vi "StartupWizard.vi"() -> (0 "Exit?":bool)   [LabVIEW 2017]
uses:
  Projekt-RubikLibrary/RubikLibrary.lvlib
  Projekt-RubikLibrary/ServoEnumControl.ctl
  Projekt-RubikLibrary/ServoAbsAngleControl.ctl
panel:
  in  "Tab Control":T1(tab)
  in  "Cancel Tab1":bool
  in  "Next Tab1":bool
  in  "Cancel Tab2":bool
  in  "Back Tab2":bool
  in  "Next Tab2":bool
  in  "Next Tab3":bool
  in  "Back Tab3":bool
  in  "Cancel Tab3":bool
  in  "Cancel Tab4":bool
  in  "Back Tab4":bool
  in  "Next Tab4":bool
  in  "Back Tab5":bool
  in  "Exit":bool
  in  "Cancel Tab5":bool
  # "Start Rubik's Cube Init"
  # "Turn Front Servo to -90° (horizontal), Left and Right Servos to 0° (vertical)\n\nClick \"Do&Next >\" or Return key"
  # "Grip Left"
  # "Left Grip will close and hold the cube. \n\nClick \"Next >\" or Return key"
  # "Grip Right"
  # "Right Grip will close and hold the cube. \n\nClick \"Next >\" or Return key"
  # "Grip Front"
  # "Front Grip will close and hold the cube. \n\nClick \"Next >\" or Return key"
  # "Startup Finished?"
  # "Either\nclick \"< Back\" to go back,\nclick \"Cancel\" to abort Startup.\nclick \"Exit\" to succesfully terminate Startup."
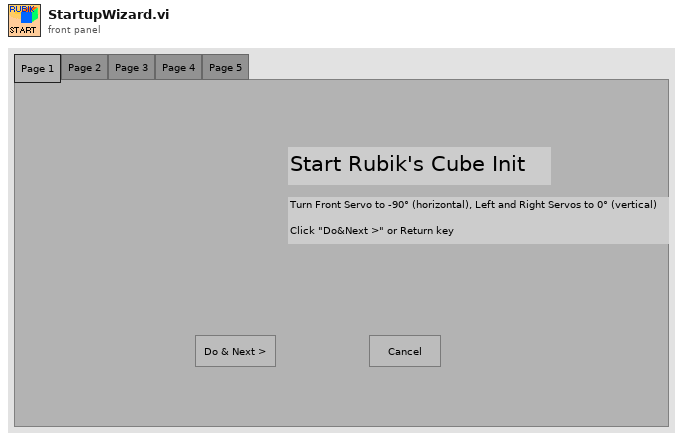
[diagram p1: front panel]
types:
  T1 = enum32{"Page 1", "Page 2", "Page 3", "Page 4", "Page 5"}
  T2 = typedef "RubikLibrary.lvlib/ServoEnumControl.ctl" = enum16{"Left Servo", "Front Servo", "Right Servo"}
  T3 = typedef "RubikLibrary.lvlib/ServoAbsAngleControl.ctl" = enum16{"-90°", "0°", "+90°"}
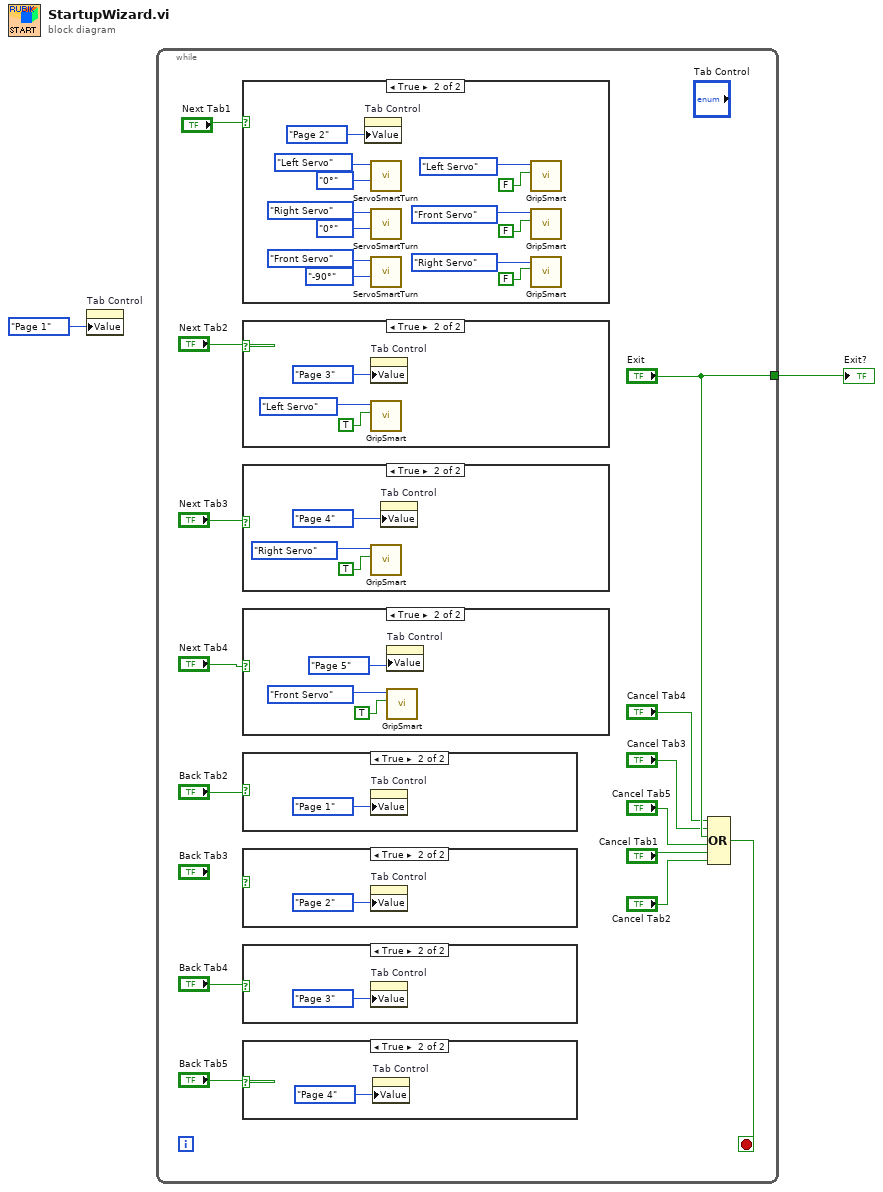
[diagram p0: block diagram]
diagram:
  n1 = property on="Tab Control" class="TabCtl (strict)"("Value"=enum32{"Page 1", "Page 2", "Page 3"}."Page 1" ("Tab Control")) -> ()  [unwired: 2 in, 2 out]
  n2 = while {
    tunnel: ["Exit"] -> w1
    stop <- w14 stop-if-true
    n3 = case shown="True" "Next Tab1" {
      frame False {
      }
      frame True {
        n4 = property on="Tab Control" class="TabCtl (strict)"("Value"=enum32{"Page 1", "Page 2", "Page 3"}."Page 2" ("Tab Control")) -> ()  [unwired: 2 in, 2 out]
        n5 = call "ServoSmartTurn.vi"("Turn to (in)"=ServoAbsAngleControl."0°", "Servo"=ServoEnumControl."Left Servo") -> ()  [unwired: 8 in, 2 out]
        n6 = call "ServoSmartTurn.vi"("Turn to (in)"=ServoAbsAngleControl."0°", "Servo"=ServoEnumControl."Right Servo") -> ()  [unwired: 8 in, 2 out]
        n7 = call "ServoSmartTurn.vi"("Turn to (in)"=ServoAbsAngleControl."-90°", "Servo"=ServoEnumControl."Front Servo") -> ()  [unwired: 8 in, 2 out]
        n8 = call "GripSmart.vi"("Turn to (in)"=FALSE, "Servo"=ServoEnumControl."Left Servo") -> ()  [unwired: 8 in, 2 out]
        n9 = call "GripSmart.vi"("Turn to (in)"=FALSE, "Servo"=ServoEnumControl."Front Servo") -> ()  [unwired: 8 in, 2 out]
        n10 = call "GripSmart.vi"("Turn to (in)"=FALSE, "Servo"=ServoEnumControl."Right Servo") -> ()  [unwired: 8 in, 2 out]
      }
    }
    n11 = case shown="True" "Next Tab2" {
      frame False {
      }
      frame True {
        n12 = property on="Tab Control" class="TabCtl (strict)"("Value"=enum32{"Page 1", "Page 2", "Page 3"}."Page 3" ("Tab Control")) -> ()  [unwired: 2 in, 2 out]
        n13 = call "GripSmart.vi"("Turn to (in)"=TRUE, "Servo"=ServoEnumControl."Left Servo") -> ()  [unwired: 8 in, 2 out]
      }
    }
    n14 = case shown="True" "Next Tab3" {
      frame False {
      }
      frame True {
        n15 = call "GripSmart.vi"("Turn to (in)"=TRUE, "Servo"=ServoEnumControl."Right Servo") -> ()  [unwired: 8 in, 2 out]
        n16 = property on="Tab Control" class="TabCtl (strict)"("Value"=T1."Page 4" ("Tab Control")) -> ()  [unwired: 2 in, 2 out]
      }
    }
    n17 = case shown="True" "Next Tab4" {
      frame False {
      }
      frame True {
        n18 = property on="Tab Control" class="TabCtl (strict)"("Value"=T1."Page 5" ("Tab Control")) -> ()  [unwired: 2 in, 2 out]
        n19 = call "GripSmart.vi"("Turn to (in)"=TRUE, "Servo"=ServoEnumControl."Front Servo") -> ()  [unwired: 8 in, 2 out]
      }
    }
    n20 = case shown="True" "Back Tab2" {
      frame False {
      }
      frame True {
        n21 = property on="Tab Control" class="TabCtl (strict)"("Value"=enum32{"Page 1", "Page 2", "Page 3"}."Page 1" ("Tab Control")) -> ()  [unwired: 2 in, 2 out]
      }
    }
    n22 = case shown="True" {
      selector: _ -> [_ _]
      frame False {
      }
      frame True {
        n23 = property on="Tab Control" class="TabCtl (strict)"("Value"=enum32{"Page 1", "Page 2", "Page 3"}."Page 2" ("Tab Control")) -> ()  [unwired: 2 in, 2 out]
      }
    }
    n24 = case shown="True" "Back Tab4" {
      frame False {
      }
      frame True {
        n25 = property on="Tab Control" class="TabCtl (strict)"("Value"=T1."Page 3" ("Tab Control")) -> ()  [unwired: 2 in, 2 out]
      }
    }
    n26 = case shown="True" "Back Tab5" {
      frame False {
      }
      frame True {
        n27 = property on="Tab Control" class="TabCtl (strict)"("Value"=T1."Page 4" ("Tab Control")) -> ()  [unwired: 2 in, 2 out]
      }
    }
    n28 = Compound Arithmetic op=OR("Cancel Tab4", "Cancel Tab3", "Exit", "Cancel Tab5", "Cancel Tab1", "Cancel Tab2") -> (w14:bool)
  }
  "Exit?" <- w1
